vi "Example - Syslog Collector.vi"() -> (11 "Log File":path=path "c:/syslog.txt")   [LabVIEW 2016, in "Logger.syslog.lvclass"]
doc: "This VI illustrates using the Syslog reference design library to implement a Syslog collector application."
uses:
  Logger.syslog.lvclass
  <vilib>/NI/syslog/_subVIs/TypeDefs/syslog_message_cluster.ctl
  <vilib>/NI/syslog/_subVIs/TypeDefs/syslog_facility_codes.ctl
  <vilib>/NI/syslog/_subVIs/TypeDefs/syslog_severity_codes.ctl
panel:
  out "Collector IP Address":string
  in  "Tab Control":enum32{"Syslog Collector", "Log File"}(tab)
  out "Messages Received":string
  out "Syslog Message":T1={"Facility Code"=enum."user", "Severity Code"=enum."emergency", "Time Stamp"=timestamp(0 s since 1904-01-01), "Hostname"="", "Message Tag"="", "Message Content"=""} {"Time Stamp" format="%<%I:%M:%S %p\n%m/%d>T"}
  out "Content":string
  in  "stop":bool
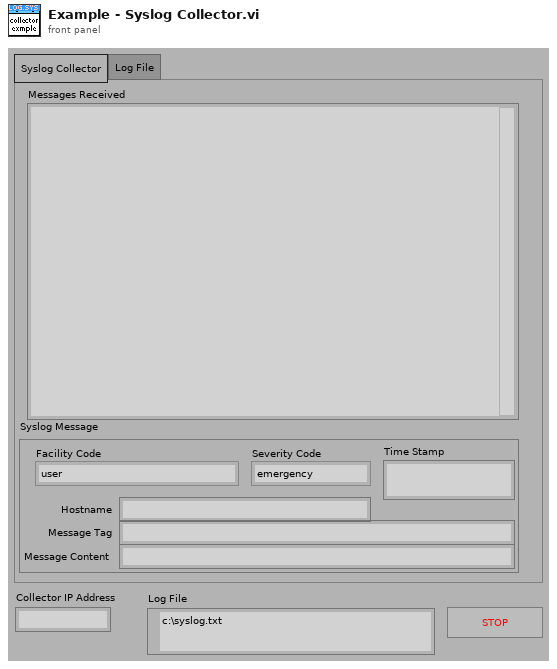
[diagram p1: front panel]
types:
  T1 = typedef "syslog_message_cluster.ctl" = cluster{"Facility Code":T2, "Severity Code":T3, "Time Stamp":timestamp, "Hostname":string, "Message Tag":string, "Message Content":string}
  T2 = typedef "syslog_facility_codes.ctl" = enum16{"kernel", "user", "mail", "system daemons", "security/authorization", "syslogd", "line printer", "network news", "uucp", "clock daemon", "security/authorization (alternate)", "FTP daemon", "NTP subsystem", "log audit", "log alert", "clock daemon (alternate)", "local use 0", "local use 1", "local use 2", "local use 3", "local use 4", "local use 5", "local use 6", "local use 7"}
  T3 = typedef "syslog_severity_codes.ctl" = enum16{"emergency", "alert", "critical", "error", "warning", "notice", "info", "debug"}
  T4 = enum16{"open", "replace", "create", "open or create", "replace or create", "replace or create with confirmation"}
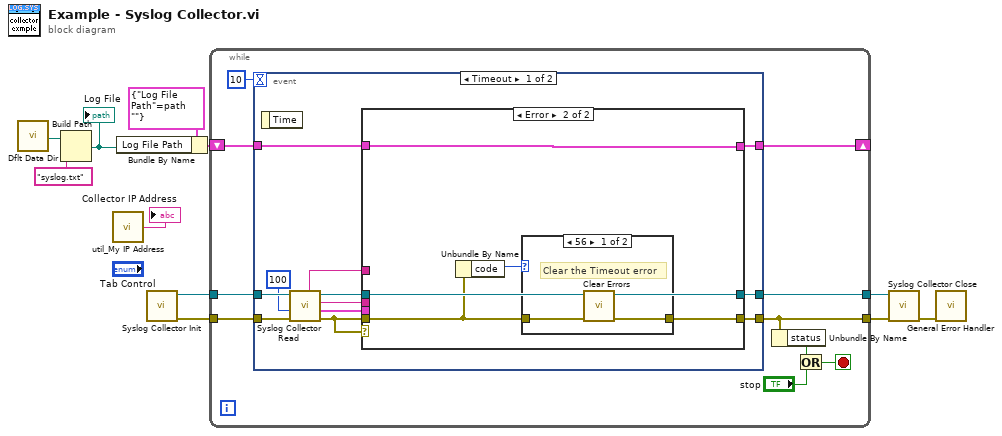
[diagram p0: block diagram]
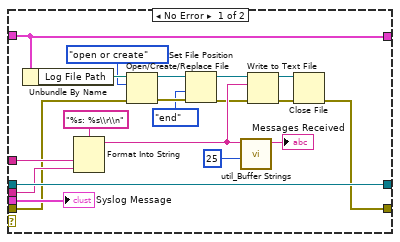
[diagram p2: hidden frame]
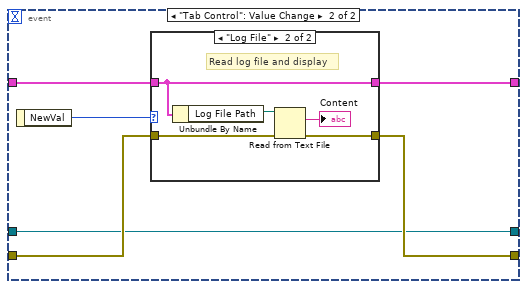
[diagram p4: hidden frame]
diagram:
  n1 = call <vilib>:"Dflt Data Dir.vi"() -> ("App:Default Data Directory"=w3:path)
  n2 = Build Path(base path=w3, name or relative path="syslog.txt") -> (appended path=w1:path)
  "Log File" <- w1
  n3 = call <vilib>:"util_My IP Address.vi"() -> ("IP Address"=→"Collector IP Address":string)  [unwired: 1 in]
  n4 = Bundle By Name(cluster=cluster{"Log File Path":path} {"Log File Path"=path ""} ("Cluster"), "Log File Path"=w1) -> (w9:cluster{"Log File Path":path})
  n5 = call <vilib>:"Syslog Collector Init.vi"() -> ("error out"=w10:errorcluster, "Syslog Collector Ref"=w11:refnum<k16>)  [unwired: 10 in]
  n6 = while {
    tunnel: w11 -> [w20]
    tunnel: w10 -> [w21]
    tunnel: [w19] -> w7
    shift-right: [w18] -> _
    shift-left: w9 -> [w16]
    tunnel: [w15] -> w5
    stop <- w12 stop-if-true
    n7 = event shown="[0] Timeout" {
      selector: _ -> [_ _]
      dyn-events: _ -> [_ _]
      timeout: 10 -> [_ _]
      tunnel: w21 -> [w33 w65]
      tunnel: w20 -> [w32 w62]
      tunnel: [w30 w62] -> w19
      tunnel: [w29 w63] -> w18
      tunnel: [w27 w64] -> w15
      tunnel: w16 -> [w23 w66]
      event Timeout {
        n8 = event-data() -> ()  [unwired: 1 in, 1 out]
        n9 = call <vilib>:"Syslog Collector Read.vi"("error in"=w33, "timeout ms (1000)"=100, "Syslog Collector Ref"=w32) -> ("error out"=w28:errorcluster, "syslog message cluster"=w24:T1, "syslog message"=w31:string, "Syslog Collector Ref"=w25:refnum<k16>, "syslog client address"=w26:string)  [unwired: 4 in]
        n10 = case shown="Error" w28 {
          tunnel: w31 -> [w44 _]
          tunnel: [w53 w58] -> w30
          tunnel: w25 -> [w53 w58]
          tunnel: w23 -> [w51 w57]
          tunnel: [w51 w57] -> w29
          tunnel: [w34 w56] -> w27
          tunnel: w28 -> [w35 w55]
          tunnel: w26 -> [w45 _]
          tunnel: w24 -> [w48 _]
          frame No Error {
            n11 = Unbundle By Name(w51) -> ("Log File Path"=w52:path)
            n12 = Format Into String(format string="%s: %s\\r\\n" ("string"), w45, w44) -> (resulting string=w47:string)  [unwired: 2 in, 1 out]
            n13 = Open/Create/Replace File(file path (use dialog)=w52, error in=w35, operation (0:open)=T4."open or create") -> (refnum out=w40:refnum<file>, error out=w41:errorcluster)  [unwired: 3 in, 1 out]
            n14 = Set File Position(refnum=w40, from (0:start)=enum16{"start", "end", "current"}."end", error in=w41) -> (refnum out=w39:refnum<file>, error out=w42:errorcluster)  [unwired: 1 in]
            n15 = call <vilib>:"util_Buffer Strings.vi"("Number of Strings to Buffer"=u8 25, "New String"=w47) -> ("Buffered String Series"=→"Messages Received":string)  [unwired: 9 in]
            n16 = Write to Text File(file (use dialog)=w39, text=w47, error in=w42) -> (refnum out=w37:refnum<file>, error out=w36:errorcluster)  [unwired: 1 in, 1 out]
            n17 = Close File(refnum=w37, error in=w36) -> (error out=w34:errorcluster)  [unwired: 1 out]
            "Syslog Message" <- w48
          }
          frame Error {
            n18 = Unbundle By Name(w55) -> ("code"=w54:i32)
            n19 = case shown="56" w54 {
              tunnel: w55 -> [w60 w61]
              tunnel: [w59 w61] -> w56
              frame 56 {
                # "Clear the Timeout error"
                n20 = call <vilib>:"Clear Errors.vi"("error in (no error)"=w60) -> ("error out"=w59:errorcluster)  [unwired: 5 in, 1 out]
              }
              frame Default {
              }
            }
          }
        }
      }
      event "Tab Control": Value Change {
        n21 = event-data() -> ("NewVal"=w67:enum32{"Syslog Collector", "Log File"})  [unwired: 1 in]
        n22 = case shown="\"Log File\"" w67 {
          tunnel: w66 -> [w68 w70]
          tunnel: w65 -> [w69 w72]
          tunnel: [w69 w71] -> w64
          tunnel: [w68 w70] -> w63
          frame "Syslog Collector", Default {
          }
          frame "Log File" {
            # "Read log file and display"
            n23 = Unbundle By Name(w70) -> ("Log File Path"=w74:path)
            n24 = Read from Text File(file (use dialog)=w74, error in=w72) -> (text=→"Content":string, error out=w71:errorcluster)  [unwired: 2 in, 2 out]
          }
        }
      }
    }
    n25 = Unbundle By Name(w15) -> ("status"=w14:bool)
    n26 = Or(x=w14, y="stop") -> (x .or. y?=w12:bool)
  }
  n27 = call <vilib>:"Syslog Collector Close.vi"("error in"=w5, "Syslog Collector Ref"=w7) -> ("error out"=w4:errorcluster)  [unwired: 9 in]
  n28 = call <vilib>:"General Error Handler.vi"("error in (no error)"=w4) -> ()  [unwired: 10 in, 5 out]
